vi "exicute_insert_query.vi"(11 "result string":string) -> (0 "error out":errorcluster)   [LabVIEW 2023]
uses:
  <vilib>/addons/database/Auxilliary.llb/DB Tools Cursor Type.ctl
  <vilib>/addons/database/Connection.llb/DB Tools Open Connec (Path).vi
  <vilib>/addons/database/Connection.llb/Conn Execute.vi
  <vilib>/addons/database/Recordset.llb/Rec Destroy - Connection.vi
  <vilib>/addons/database/NI_Database_API.lvlib
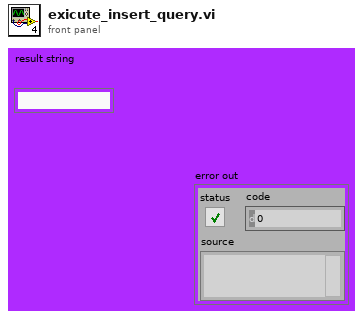
[diagram p1: front panel]
types:
  T1 = typedef "NI_Database_API.lvlib/DB Tools Cursor Type.ctl" = enum16{"forward-only", "keyset", "dynamic", "static"}
  T2 = typedef "NI_Database_API.lvlib/Conn ObjectReference.ctl" = refnum<k1>
  T3 = typedef "NI_Database_API.lvlib/Rec ObjectReference.ctl" = refnum<k1>
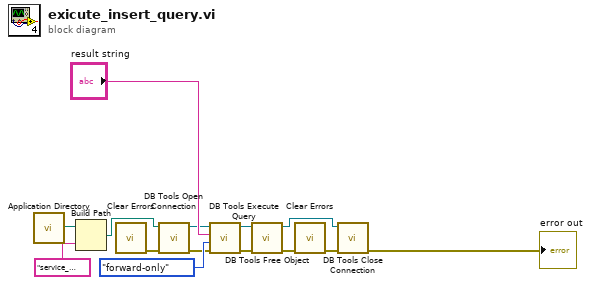
[diagram p0: block diagram]
diagram:
  n1 = call <vilib>:"Application Directory.vi"() -> ("Application Directory"=w6:path)
  n2 = Build Path(base path=w6, name or relative path="service_calls_entries.udl") -> (appended path=w9:path)
  n3 = call <vilib>:"Clear Errors.vi"() -> ("error out"=w8:errorcluster)  [unwired: 6 in, 1 out]
  n4 = call-poly <vilib>:"DB Tools Open Connection.vi"("error in (no error)"=w8, "connection information"=w9) -> ("error out"=w2:errorcluster, "connection reference"=w1:T2)  [unwired: 6 in]
  n5 = call-poly <vilib>:"DB Tools Execute Query.vi"("error in (no error)"=w2, "cursor type"=DB_Tools_Cursor_Type."forward-only", "SQL query"="result string", "connection reference"=w1) -> ("error out"=w12:errorcluster, "recordset reference"=w11:T3)  [unwired: 4 in]
  n6 = call-poly <vilib>:"DB Tools Free Object.vi"("error in (no error)"=w12, "recordset reference"=w11) -> ("error out"=w5:errorcluster, "connection reference"=w3:T2)  [unwired: 8 in]
  n7 = call <vilib>:"Clear Errors.vi"("error in (no error)"=w5) -> ("error out"=w4:errorcluster)  [unwired: 5 in, 1 out]
  n8 = call <vilib>:"DB Tools Close Connection.vi"("error in (no error)"=w4, "connection reference"=w3) -> ("error out"=→"error out":errorcluster)  [unwired: 5 in]
